vi "GetStraight EdgeResultValue.vi"(8 "error in (no error)":errorcluster, 9 "data":T1(array[cluster]), 11 "Analysis_Find Straight Edge_Parameter":T2={"ROI Descriptor"={"Global Rectangle"=[], "Contours"=[]}, "Number of Matches Requested"=1, "Edge Info Size"=0, "Options"={"Search Direction"=0, "Edge Options"={"Edge Polarity"=0, "Kernel Size"=4, "Width"=3, "Minimum Edge Strength"=1024.0, "Interpolation Type"=enum."Zero Order", "Data Processing Method"=enum."Median"}, "Show Search Area"=FALSE, "Show Search Lines"=FALSE, "Show Edges Found"=FALSE, "Show Result"=TRUE, "Search Area Color"=5, "Search Lines Color"=3, "Edge Locations Color"=50, "Result Color"=1, "Overlay Group Name"=""}, "Line Fit Options"={"Number of Lines"=0, "Type"=enum."Best Edge Rake", "Min. Score"=0.0, "Max. Score"=25.0, "Orientation"=5.0, "Angle Range"=45.0, "Angle Tolerance"=1.0, "Step Size"=7, "Min. SNR (db)"=0.0, "Min. Points (%)"=25.0, "Hough Iterations"=5}} {"Line Fit Options"."Min. Points (%)" min=0.0 max=100.0; "Line Fit Options"."Min. SNR (db)" min=0.0; "Line Fit Options"."Max. Score" min=0.0 max=1024.0; "Line Fit Options"."Min. Score" min=0.0 max=1024.0 step=1.0; "Options"."Edge Options"."Edge Polarity" items=["All Edges", "Rising Edges", "Falling Edges"]; "Options"."Edge Options"."Minimum Edge Strength" format="%.2f"; "Options"."Edge Options"."Width" step=2; "Options"."Edge Options"."Kernel Size" step=2; "Options"."Search Direction" items=["Left to Right", "Right to Left", "Top to Bottom", "Bottom to Top"]}) -> (0 "error out":errorcluster, 3 "ResultValues":string[](array[string]))   [LabVIEW 2019]
uses:
  Controls/Find Straight Edge/Analysis_Find Straight Edge_Parameter.ctl
  <vilib>/vision/Measure.llb/Edge Options.ctl
  <vilib>/vision/Measure.llb/Edge Polarity.ctl
  <vilib>/vision/Measure.llb/Straight Edge Options.ctl
  <vilib>/vision/Measure.llb/Straight Edge Process.ctl
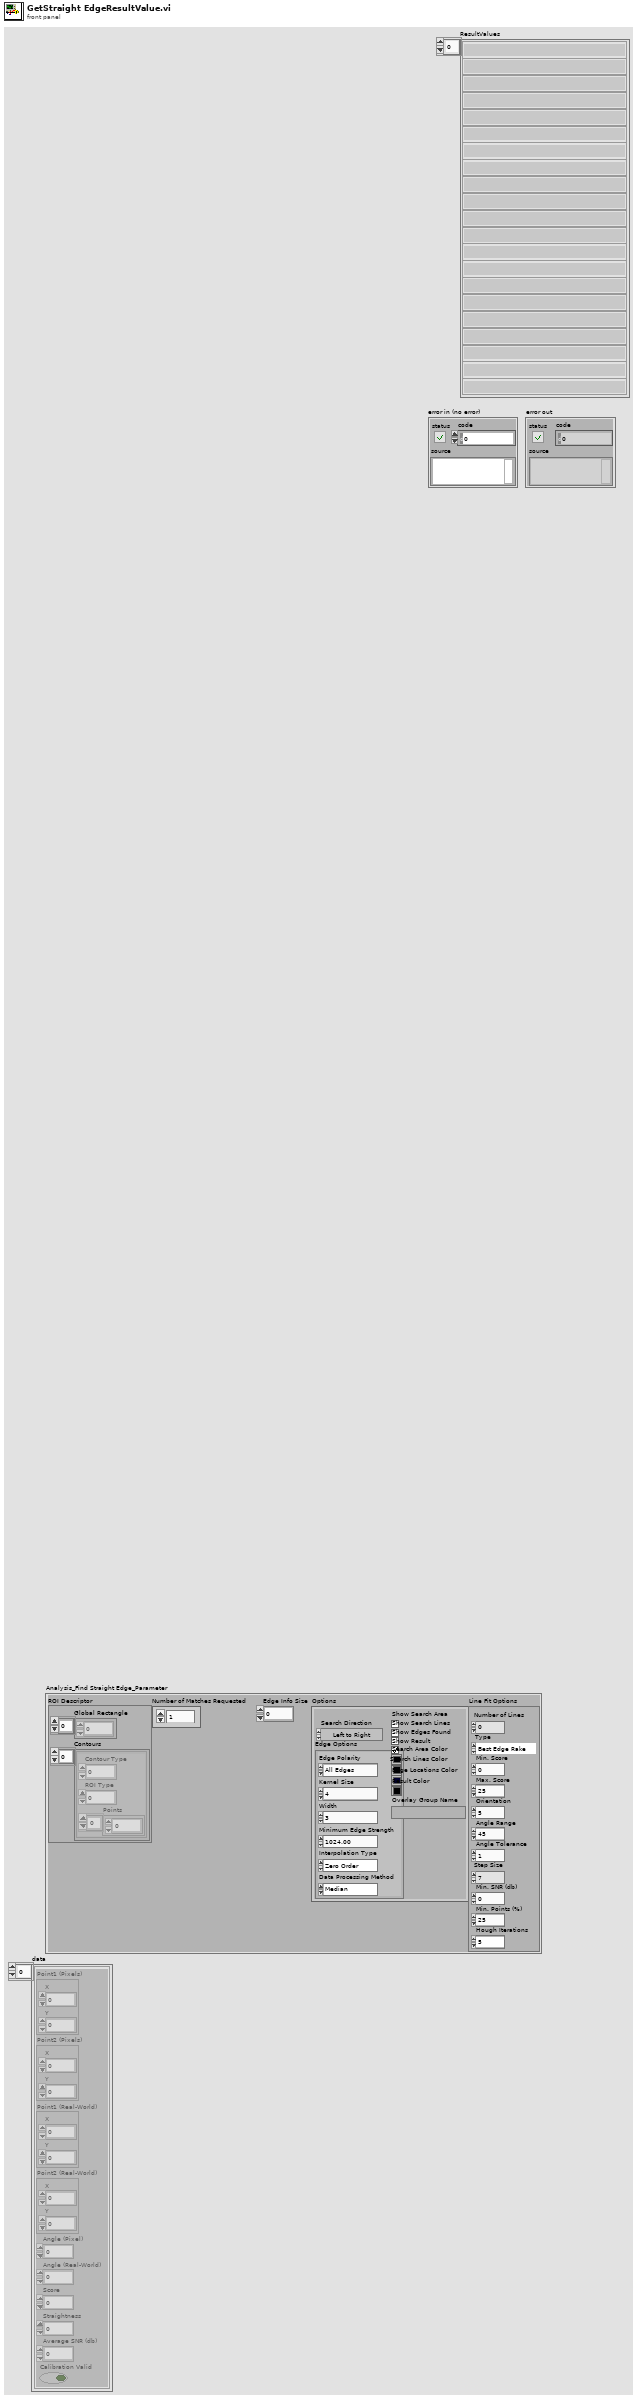
[diagram p1: front panel]
types:
  T1 = cluster{"Point1 (Pixels)":cluster{"X":sgl, "Y":sgl}, "Point2 (Pixels)":cluster{"X":sgl, "Y":sgl}, "Point1 (Real-World)":cluster{"X":sgl, "Y":sgl}, "Point2 (Real-World)":cluster{"X":sgl, "Y":sgl}, "Angle (Pixel)":dbl, "Angle (Real-World)":dbl, "Score":dbl, "Straightness":dbl, "Average SNR (db)":dbl, "Calibration Valid":bool}[]
  T2 = typedef "Analysis_Find Straight Edge_Parameter.ctl" = cluster{"ROI Descriptor":cluster{"Global Rectangle":i32[], "Contours":cluster{"Contour Type":u32, "ROI Type":u32, "Points":i32[]}[]}, "Number of Matches Requested":i32, "Edge Info Size":i32, "Options":cluster{"Search Direction":u32, "Edge Options":T3, "Show Search Area":bool, "Show Search Lines":bool, "Show Edges Found":bool, "Show Result":bool, "Search Area Color":u32, "Search Lines Color":u32, "Edge Locations Color":u32, "Result Color":u32, "Overlay Group Name":string}, "Line Fit Options":T5}
  T3 = typedef "Edge Options.ctl" = cluster{"Edge Polarity":T4, "Kernel Size":u32, "Width":u32, "Minimum Edge Strength":sgl, "Interpolation Type":enum32{"Zero Order", "Bilinear", "Quadratic", "Cubic", "Bilinear Fixed"}, "Data Processing Method":enum32{"Average", "Median"}}
  T4 = typedef "Edge Polarity.ctl" = u32
  T5 = typedef "Straight Edge Options.ctl" = cluster{"Number of Lines":i32, "Type":T6, "Min. Score":dbl, "Max. Score":dbl, "Orientation":dbl, "Angle Range":dbl, "Angle Tolerance":dbl, "Step Size":u32, "Min. SNR (db)":dbl, "Min. Points (%)":dbl, "Hough Iterations":i32}
  T6 = typedef "Straight Edge Process.ctl" = enum32{"First Edge Rake", "Best Edge Rake", "Hough Edge Rake", "First Edge Projection", "Best Edge Projection"}
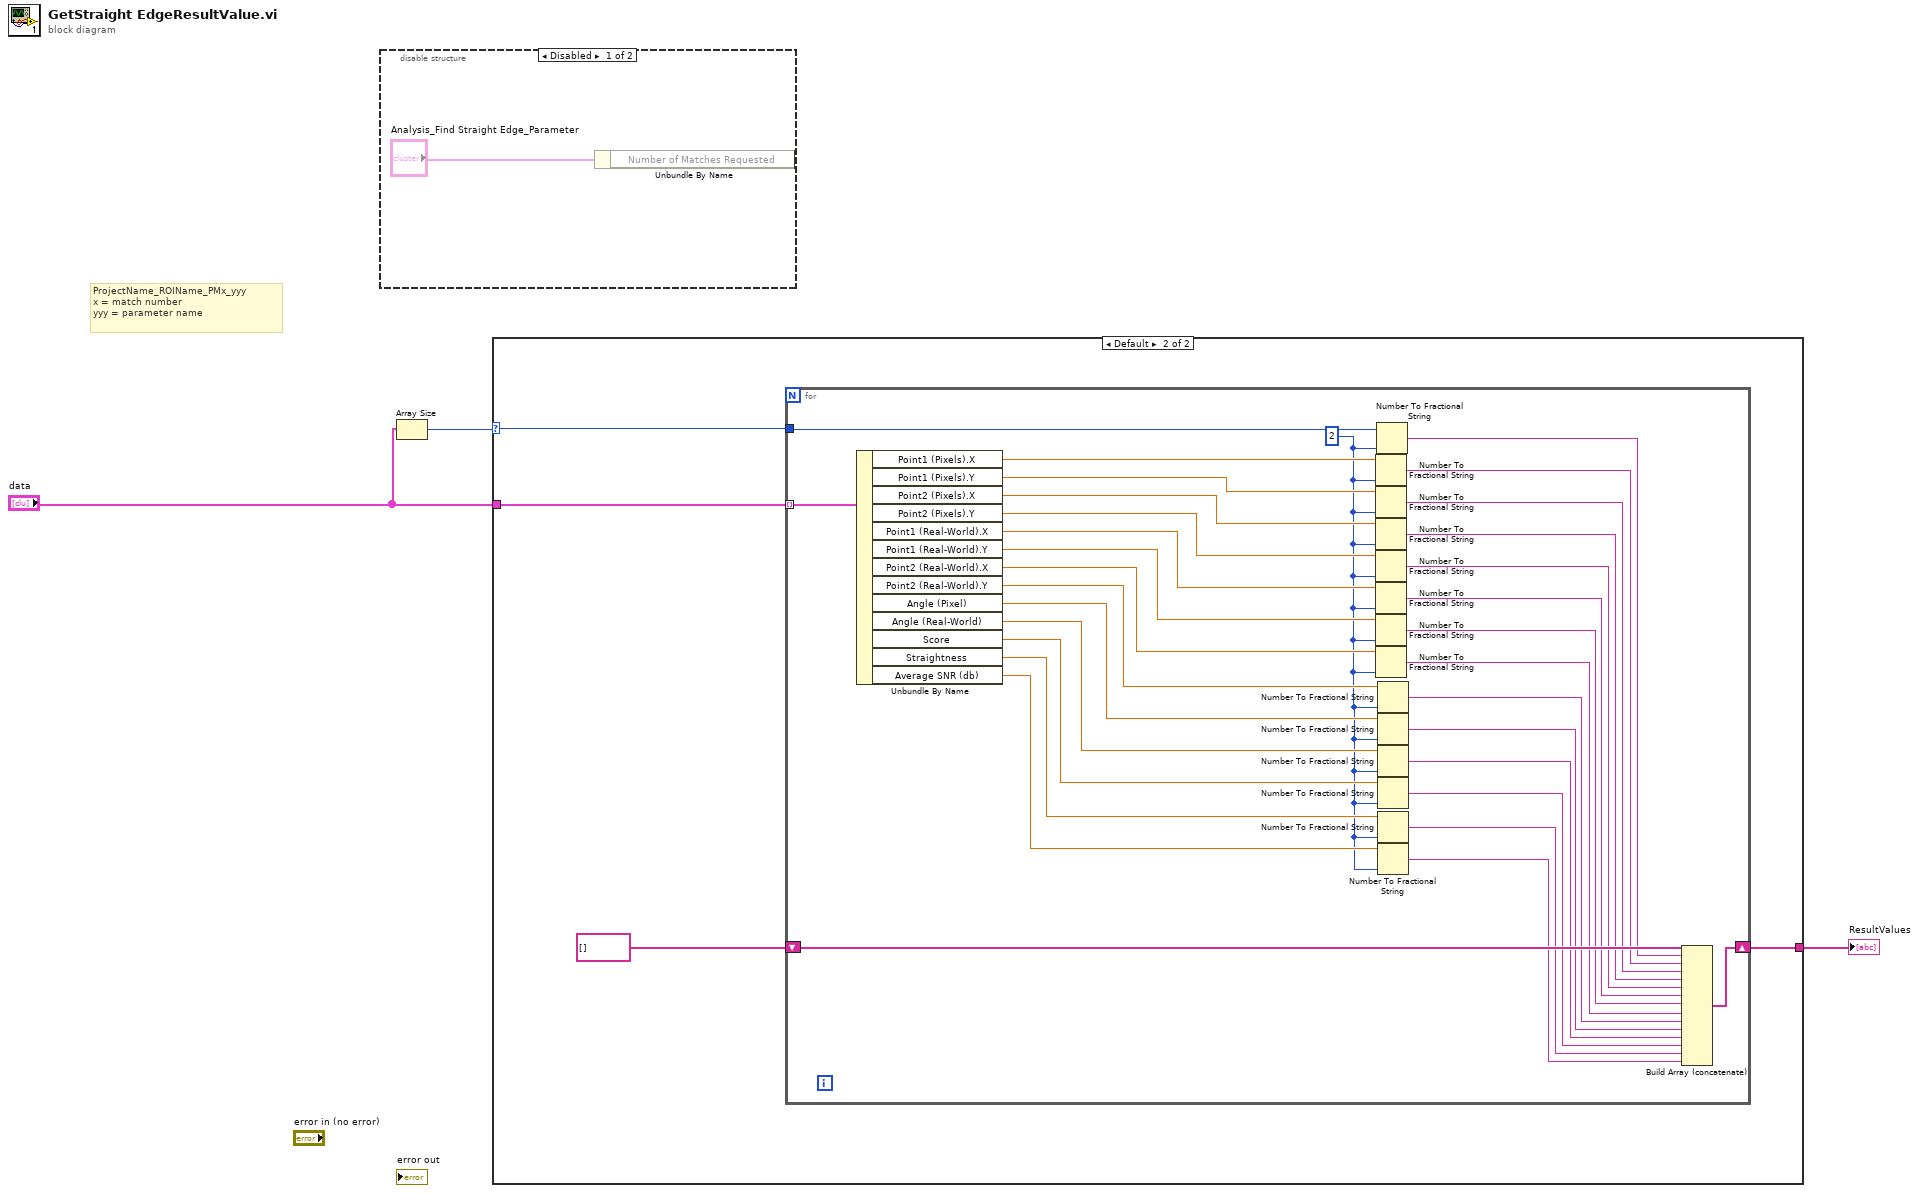
[diagram p0: block diagram]
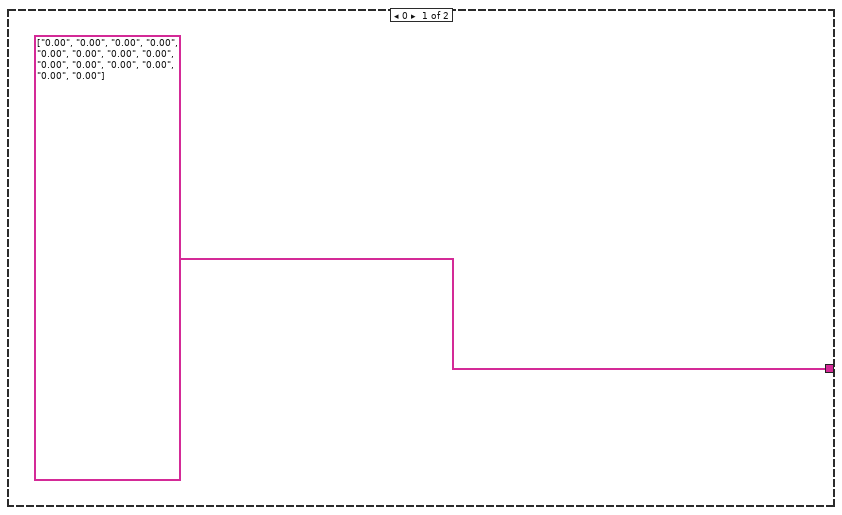
[diagram p2: hidden frame]
diagram:
  # "ProjectName_ROIName_PMx_yyy\nx = match number\nyyy = parameter name"
  n1 = disable-structure shown="Disabled" {
    frame Disabled {
      n2 = Unbundle By Name("Analysis_Find Straight Edge_Parameter") -> ()  [unwired: 1 out]
    }
    frame Enabled {
    }
  }
  n3 = Array Size(array="data") -> (size(s)=w1:i32)
  n4 = case shown="Default" w1 {
    selector: w1 -> [_ w6]
    tunnel: [string[] ["0.00", "0.00", "0.00", "0.00", "0.00", "0.00", "0.00", "0.00", "0.00", "0.00", "0.00", "0.00", "0.00", "0.00"] w8] -> w3
    tunnel: "data" -> [_ w7]
    frame 0 {
    }
    frame Default {
      n5 = for {
        shift-right: [w34] -> w8
        shift-left: string[] [] -> [w41]
        tunnel: w7 -> [w29] mode=indexing
        tunnel: w6 -> [w12]
        w11 = 2
        n6 = Unbundle By Name(w29) -> ("Point1 (Pixels).X"=w28:sgl, "Point1 (Pixels).Y"=w27:sgl, "Point2 (Pixels).X"=w26:sgl, "Point2 (Pixels).Y"=w25:sgl, "Point1 (Real-World).X"=w24:sgl, "Point1 (Real-World).Y"=w23:sgl, "Point2 (Real-World).X"=w22:sgl, "Point2 (Real-World).Y"=w21:sgl, "Angle (Pixel)"=w20:dbl, "Angle (Real-World)"=w19:dbl, "Score"=w18:dbl, "Straightness"=w14:dbl, "Average SNR (db)"=w13:dbl)
        n7 = Number To Fractional String(number=w28, precision (6)=w11) -> (F-format string=w40:string)  [unwired: 2 in]
        n8 = Number To Fractional String(number=w27, precision (6)=w11) -> (F-format string=w39:string)  [unwired: 2 in]
        n9 = Number To Fractional String(number=w26, precision (6)=w11) -> (F-format string=w38:string)  [unwired: 2 in]
        n10 = Number To Fractional String(number=w25, precision (6)=w11) -> (F-format string=w37:string)  [unwired: 2 in]
        n11 = Number To Fractional String(number=w24, precision (6)=w11) -> (F-format string=w36:string)  [unwired: 2 in]
        n12 = Number To Fractional String(number=w23, precision (6)=w11) -> (F-format string=w35:string)  [unwired: 2 in]
        n13 = Number To Fractional String(number=w22, precision (6)=w11) -> (F-format string=w17:string)  [unwired: 2 in]
        n14 = Number To Fractional String(number=w12, precision (6)=w11) -> (F-format string=w10:string)  [unwired: 2 in]
        n15 = Number To Fractional String(number=w21, precision (6)=w11) -> (F-format string=w33:string)  [unwired: 2 in]
        n16 = Number To Fractional String(number=w20, precision (6)=w11) -> (F-format string=w32:string)  [unwired: 2 in]
        n17 = Number To Fractional String(number=w19, precision (6)=w11) -> (F-format string=w31:string)  [unwired: 2 in]
        n18 = Number To Fractional String(number=w18, precision (6)=w11) -> (F-format string=w30:string)  [unwired: 2 in]
        n19 = Number To Fractional String(number=w14, precision (6)=w11) -> (F-format string=w16:string)  [unwired: 2 in]
        n20 = Number To Fractional String(number=w13, precision (6)=w11) -> (F-format string=w15:string)  [unwired: 2 in]
        n21 = Build Array (concatenate)(w41, w10, w40, w39, w38, w37, w36, w35, w17, w33, w32, w31, w30, w16, w15) -> (w34:string[])
      }
    }
  }
  "ResultValues" <- w3
